vi "Initialization VI.vi"(8 "error in (no error)":errorcluster, 10 "Custom XML":string, 11 "Device Item Ref in":T1 format="%.0x") -> (0 "error out":errorcluster, 3 "Device Item Ref out":T1 format="%.0x")   [LabVIEW 2019, in "Displacement Measurement CD System Explorer.lvlib"]
uses:
  Displacement Measurement CD System Explorer.lvlib
  <vilib>/NI VeriStand/Custom Device API/Custom Device Item Ref.ctl
  <vilib>/NI VeriStand/Custom Device API/Custom Device Channel.ctl
  <vilib>/NI VeriStand/Custom Device API/Custom Device Channel Type.ctl
  <vilib>/NI VeriStand/Custom Device API/Custom Device API.lvlib
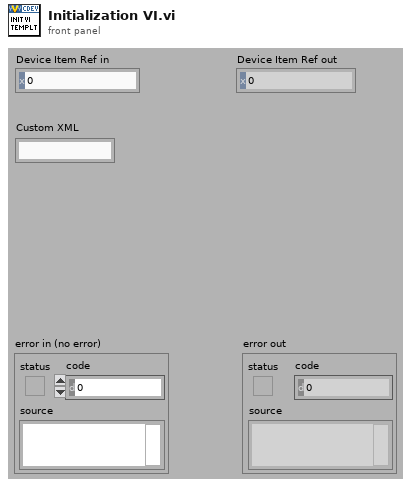
[diagram p1: front panel]
types:
  T1 = typedef "Custom Device API.lvlib/Custom Device Item Ref.ctl" = u64
  T2 = typedef "Custom Device API.lvlib/Custom Device Channel.ctl" = cluster{"Type":T3, "Units":string, "Default Value":dbl, "Faultable":bool, "Scalable":bool}
  T3 = typedef "Custom Device API.lvlib/Custom Device Channel Type.ctl" = enum16{"Input", "Output"}
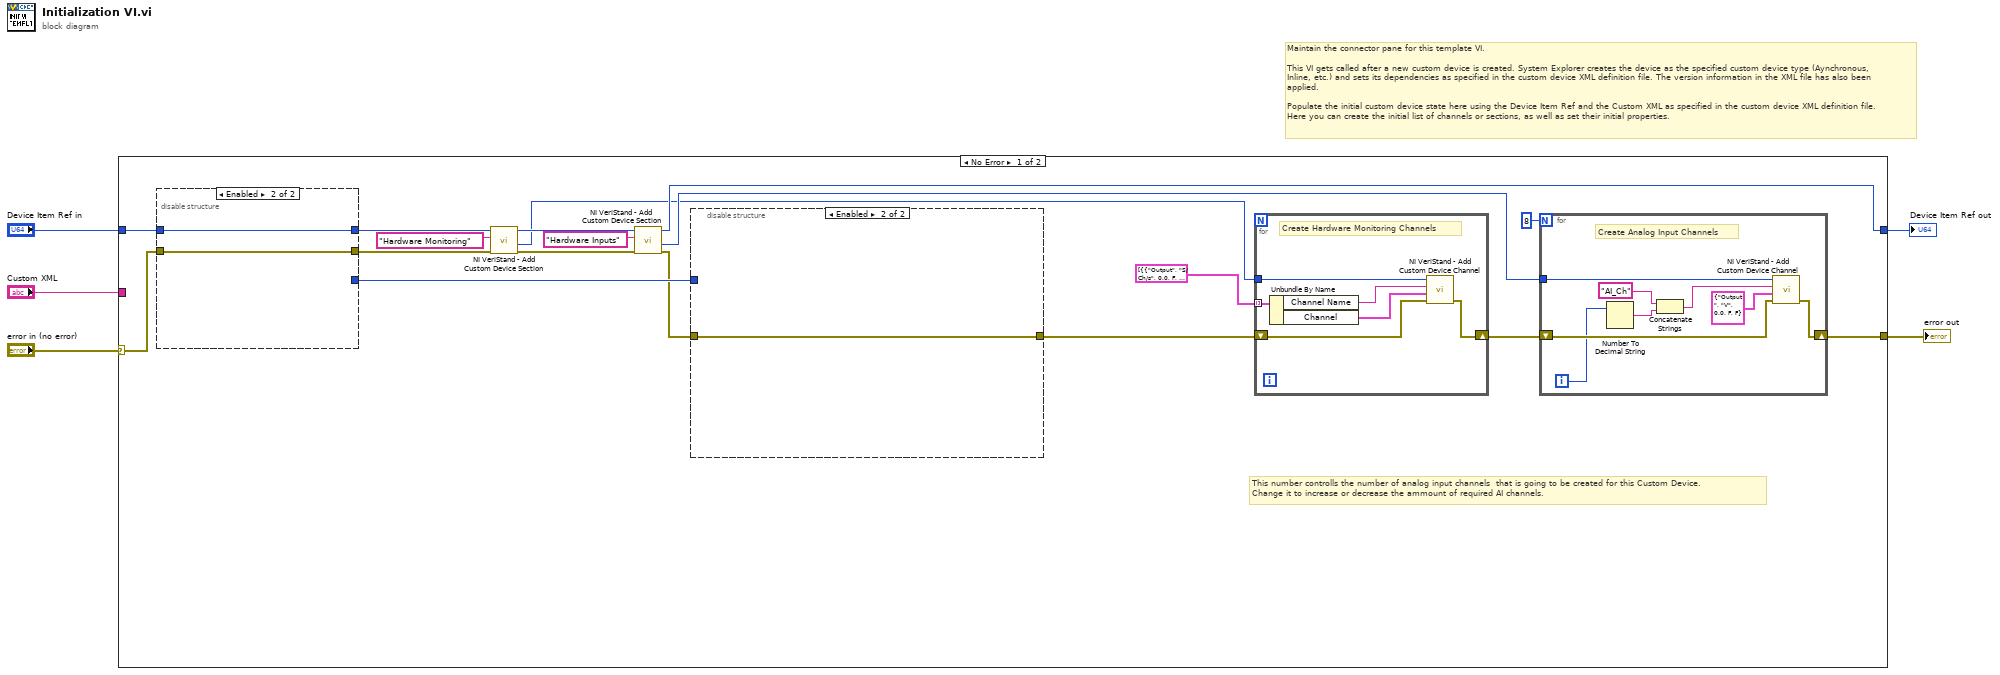
[diagram p0: block diagram]
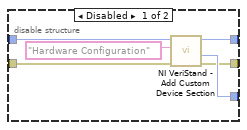
[diagram p2: hidden frame]
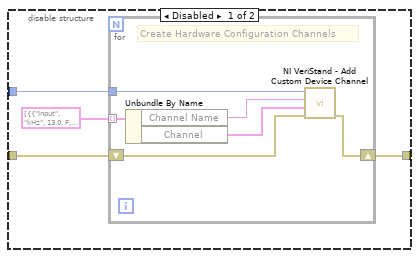
[diagram p3: hidden frame]
diagram:
  # "Maintain the connector pane for this template VI.\n\nThis VI gets called after a new custom device is created. System Explorer creates the device as the specified custom device type (Aynchronous, Inline, etc.) and sets its dependencies as specified in the custom device XML definition file. The version information in the XML file has also been applied.\n\nPopulate the initial custom device state here using the Device Item Ref and the Custom XML as specified in the custom device XML definition file. Here you can create the initial list of channels or sections, as well as set their initial properties."
  n1 = case shown="No Error" "error in (no error)" {
    selector: "error in (no error)" -> [w21 w58]
    tunnel: [w8 w58] -> w2
    tunnel: [w16 w57] -> w1
    tunnel: "Device Item Ref in" -> [w22 w57]
    tunnel: "Custom XML" -> [_ _]
    frame No Error {
      # "This number controlls the number of analog input channels  that is going to be created for this Custom Device.\nChange it to increase or decrease the ammount of required AI channels."
      n2 = disable-structure shown="Enabled" {
        disable-tunnel: w22 -> [w29 w30]
        disable-tunnel: w21 -> [w28 w31]
        disable-tunnel: [w27 _] -> w20
        disable-tunnel: [w26 w30] -> w14
        disable-tunnel: [w25 w31] -> w13
        frame Disabled {
          n3 = call <vilib>:"NI VeriStand - Add Custom Device Section.vi"("error in (no error)"=w28, "Section Name"="Hardware Configuration", "Parent Ref in"=w29) -> ("error out"=w25:errorcluster, "Section Ptr"=w27:T1, "Parent Ref out"=w26:T1)  [unwired: 5 in, 1 out]
        }
        frame Enabled {
        }
      }
      n4 = call <vilib>:"NI VeriStand - Add Custom Device Section.vi"("error in (no error)"=w13, "Section Name"="Hardware Monitoring", "Parent Ref in"=w14) -> ("error out"=w11:errorcluster, "Section Ptr"=w9:T1, "Parent Ref out"=w12:T1)  [unwired: 5 in, 1 out]
      n5 = call <vilib>:"NI VeriStand - Add Custom Device Section.vi"("error in (no error)"=w11, "Section Name"="Hardware Inputs", "Parent Ref in"=w12) -> ("error out"=w19:errorcluster, "Section Ptr"=w18:T1, "Parent Ref out"=w16:T1)  [unwired: 5 in, 1 out]
      n6 = disable-structure shown="Enabled" {
        disable-tunnel: w20 -> [w35 _]
        disable-tunnel: w19 -> [w34 w42]
        disable-tunnel: [w33 w42] -> w6
        frame Disabled {
          n7 = for {
            tunnel: cluster{"Channel":T2, "Channel Name":string}[] [{"Channel"={"Type"=enum."Input", "Units"="kHz", "Default Value"=13.0, "Faultable"=FALSE, "Scalable"=FALSE}, "Channel Name"="Loop Rate"}, {"Channel"={"Type"=enum."Input", "Units"="S/Ch/s", "Default Value"=1000.0, "Faultable"=FALSE, "Scalable"=FALSE}, "Channel Name"="Sampling Frequency"}, {"Channel"={"Type"=enum."Input", "Units"="V", "Default Value"=-10.0, "Faultable"=FALSE, "Scalable"=FALSE}, "Channel Name"="Min. Voltage"}, {"Channel"={"Type"=enum."Input", "Units"="", "Default Value"=10.0, "Faultable"=FALSE, "Scalable"=FALSE}, "Channel Name"="Max. Voltage"}] -> [w41] mode=indexing
            tunnel: w35 -> [w40]
            shift-right: [w36] -> w33
            shift-left: w34 -> [w37]
            # "Create Hardware Configuration Channels"
            n8 = Unbundle By Name(w41) -> ("Channel Name"=w39:string, "Channel"=w38:T2)
            n9 = call <vilib>:"NI VeriStand - Add Custom Device Channel.vi"("error in (no error)"=w37, "Channel"=w38, "Channel Name"=w39, "Parent Ref in"=w40) -> ("error out"=w36:errorcluster)  [unwired: 4 in, 3 out]
          }
        }
        frame Enabled {
        }
      }
      n10 = for {
        tunnel: cluster{"Channel":T2, "Channel Name":string}[] [{"Channel"={"Type"=enum."Output", "Units"="S/Ch/s", "Default Value"=0.0, "Faultable"=FALSE, "Scalable"=FALSE}, "Channel Name"="Actual Sample Rate"}, {"Channel"={"Type"=enum."Output", "Units"="kHz", "Default Value"=0.0, "Faultable"=FALSE, "Scalable"=FALSE}, "Channel Name"="Actual Loop Rate"}] -> [w48] mode=indexing
        tunnel: w9 -> [w47]
        shift-right: [w43] -> w7
        shift-left: w6 -> [w44]
        # "Create Hardware Monitoring Channels"
        n11 = Unbundle By Name(w48) -> ("Channel Name"=w46:string, "Channel"=w45:T2)
        n12 = call <vilib>:"NI VeriStand - Add Custom Device Channel.vi"("error in (no error)"=w44, "Channel"=w45, "Channel Name"=w46, "Parent Ref in"=w47) -> ("error out"=w43:errorcluster)  [unwired: 4 in, 3 out]
      }
      n13 = for {
        N: 8 -> [_]
        tunnel: w18 -> [w56]
        shift-right: [w54] -> w8
        shift-left: w7 -> [w55]
        i -> [w52]
        # "Create Analog Input Channels"
        n14 = Number To Decimal String(number=w52) -> (decimal integer string=w50:string)  [unwired: 1 in]
        n15 = Concatenate Strings("AI_Ch" ("Channel Name"), w50) -> (w49:string)
        n16 = call <vilib>:"NI VeriStand - Add Custom Device Channel.vi"("error in (no error)"=w55, "Channel"=T2 {"Type"=enum."Output", "Units"="V", "Default Value"=0.0, "Faultable"=FALSE, "Scalable"=FALSE}, "Channel Name"=w49, "Parent Ref in"=w56) -> ("error out"=w54:errorcluster)  [unwired: 4 in, 3 out]
      }
    }
    frame Error {
    }
  }
  "error out" <- w2
  "Device Item Ref out" <- w1
